vi "PlotDrag-Get Plot At Position.vi"(0 "XYGraph in":refnum<vi>, 7 "Coords":T1, 9 "Threshold":i32=5, 11 "error in (no error)":errorcluster) -> (4 "XYGraph out":refnum<vi>, 6 "PlotNum":i32, 8 "Plot Name":string, 15 "error out":errorcluster)   [LabVIEW 2020]
uses:
  <vilib>/Utility/miscctls.llb/LVPoint32TypeDef.ctl
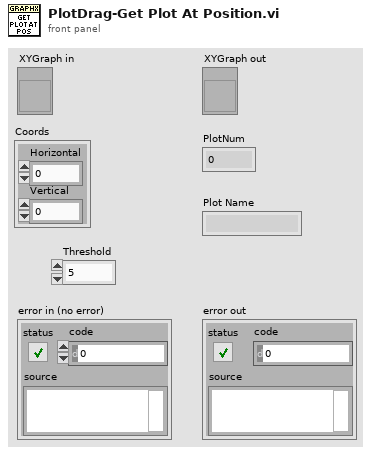
[diagram p1: front panel]
types:
  T1 = typedef "LVPoint32TypeDef.ctl" = cluster{"Horizontal":i32, "Vertical":i32}
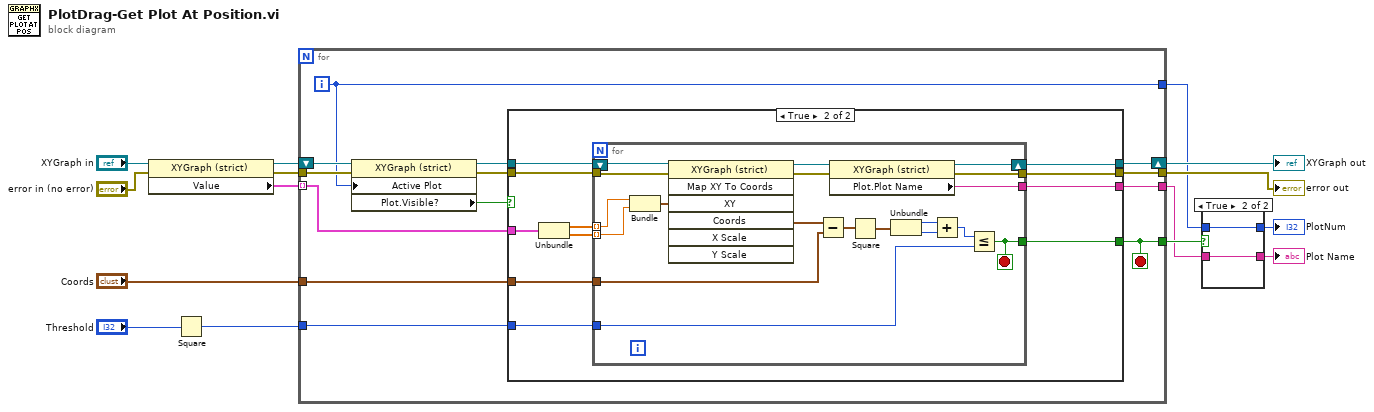
[diagram p0: block diagram]
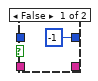
[diagram p2: hidden frame]
diagram:
  n1 = property class="XYGraph (strict)"(reference="XYGraph in", error in="error in (no error)") -> (reference out=w13:refnum<vi>, error out=w12:errorcluster, "Value"=w11:cluster{dbl[], dbl[]}[])
  n2 = Square(x="Threshold") -> (x^2=w6:i32)
  n3 = for {
    tunnel: w12 -> [w27]
    tunnel: w11 -> [w25] mode=indexing
    tunnel: [w22] -> w10
    tunnel: "Coords" -> [w20]
    tunnel: w6 -> [w19]
    shift-right: [w21] -> w9
    shift-left: w13 -> [w28]
    tunnel: [w18] -> w5
    tunnel: [w17] -> w3
    tunnel: [w16] -> w2
    i -> [w17]
    stop <- w18 stop-if-true
    n4 = property class="XYGraph (strict)"(reference=w28, error in=w27, "Active Plot"=w17) -> (reference out=w24:refnum<vi>, error out=w23:errorcluster, "Plot.Visible?"=w26:bool)
    n5 = case shown="True" w26 {
      tunnel: w25 -> [_ w41]
      tunnel: w24 -> [w30 w38]
      tunnel: w23 -> [w29 w37]
      tunnel: [_ w32] -> w18
      tunnel: [w29 w33] -> w22
      tunnel: [w30 w34] -> w21
      tunnel: w20 -> [_ w36]
      tunnel: w19 -> [_ w35]
      tunnel: [_ w31] -> w16
      frame False {
      }
      frame True {
        n6 = Unbundle(w41) -> (w40:dbl[], w39:dbl[])
        n7 = for {
          tunnel: w40 -> [w56] mode=indexing
          tunnel: w39 -> [w55] mode=indexing
          tunnel: [w60] -> w32
          tunnel: w37 -> [w58]
          tunnel: w36 -> [w53]
          tunnel: w35 -> [w48]
          tunnel: [w43] -> w33
          shift-right: [w44] -> w34
          shift-left: w38 -> [w59]
          tunnel: [w42] -> w31
          stop <- w60 stop-if-true
          n8 = Bundle(w56, w55) -> (w57:cluster{dbl, dbl})  [unwired: 1 in]
          n9 = invoke class="XYGraph (strict)" method="Map XY To Coords"(reference=w59, error in=w58, "XY"=w57) -> (reference out=w46:refnum<vi>, error out=w45:errorcluster, "Coords"=w54:T1)  [unwired: 4 in, 4 out]
          n10 = Subtract(x=w54, y=w53) -> (x-y=w52:T1)
          n11 = property class="XYGraph (strict)"(reference=w46, error in=w45) -> (reference out=w44:refnum<vi>, error out=w43:errorcluster, "Plot.Plot Name"=w42:string)
          n12 = Square(x=w52) -> (x^2=w51:T1)
          n13 = Unbundle(w51) -> ("Horizontal"=w50:i32, "Vertical"=w49:i32)
          n14 = Add(x=w50, y=w49) -> (x+y=w47:i32)
          n15 = Less Or Equal?(x=w47, y=w48) -> (x <= y?=w60:bool)
        }
      }
    }
  }
  "error out" <- w10
  "XYGraph out" <- w9
  n16 = case shown="True" w5 {
    tunnel: [-1 w63] -> w4
    tunnel: w3 -> [_ w63]
    tunnel: w2 -> [_ w62]
    tunnel: [_ w62] -> w1
    frame False {
    }
    frame True {
    }
  }
  "PlotNum" <- w4
  "Plot Name" <- w1
